vi "Update.vi"(6 "Table Name":string, 7 "condition":string, 8 "error in (no error)":errorcluster, 9 "Data List":variant, 10 "ColumnName List":variant, 11 "DataBase_SQL in":refnum<class "DataBase_SQL.lvclass">) -> (0 "error out":errorcluster, 2 "SQL Query":string, 3 "DataBase_SQL out":refnum<class "DataBase_SQL.lvclass">)   [LabVIEW 2021, in "DataBase_SQL.lvclass"]
uses:
  <userlib>/John_Lib/DataBase/DataBase_SQL/DataBase_SQL.lvclass
  <userlib>/John_Lib/DataBase/DataBase_SQL/DataBase_SQL.lvclass/DataBase_SQL.ctl
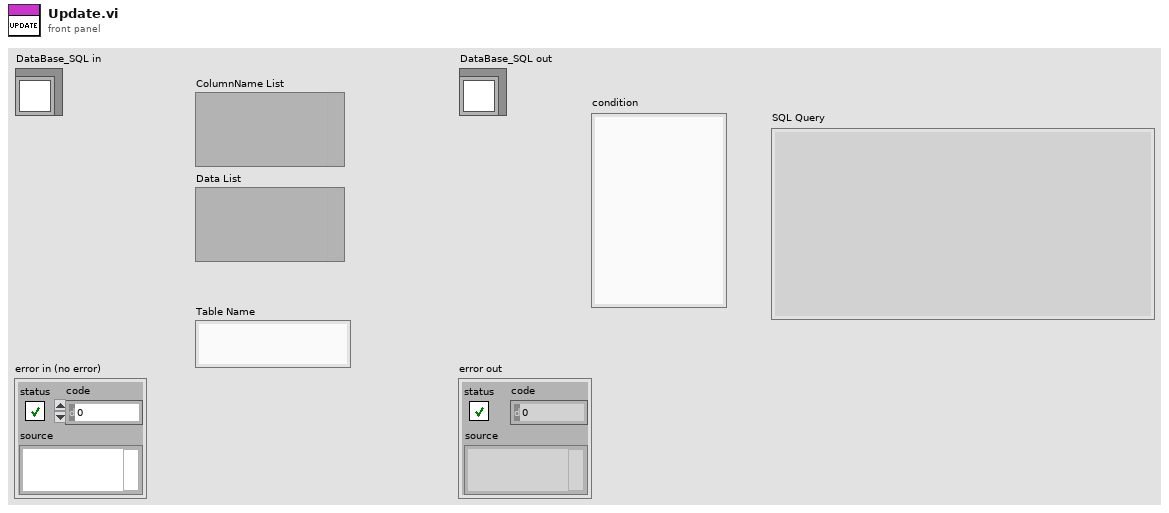
[diagram p1: front panel]
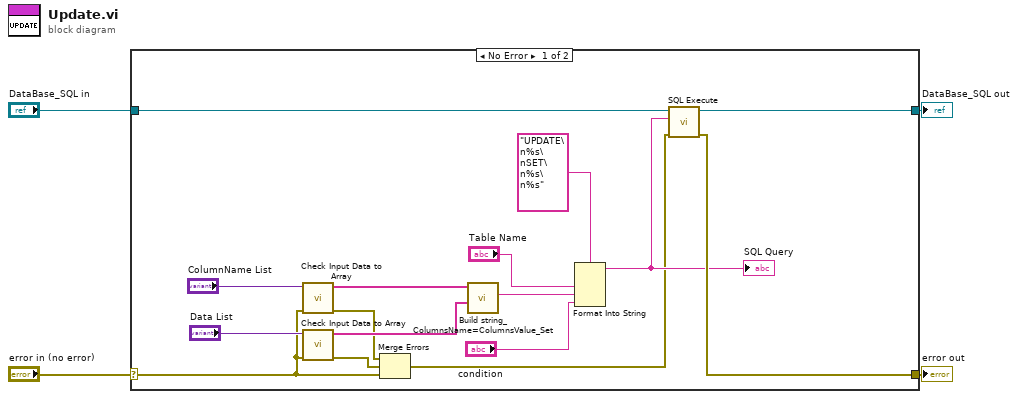
[diagram p0: block diagram]
diagram:
  n1 = case shown="No Error" "error in (no error)" {
    selector: "error in (no error)" -> [w8 w22]
    tunnel: [w16 w22] -> w3
    tunnel: [w18 w21] -> w1
    tunnel: "DataBase_SQL in" -> [w17 w21]
    frame No Error {
      n2 = call <userlib>:"Check Input Data to Array.vi"("error in (no error)"=w8, "String Array/ String"="ColumnName List") -> ("error out"=w6:errorcluster, "ColumnsNameList"=w11:string[])  [unwired: 8 in]
      n3 = call <userlib>:"Check Input Data to Array.vi"("error in (no error)"=w8, "String Array/ String"="Data List") -> ("error out"=w5:errorcluster, "ColumnsNameList"=w12:string[])  [unwired: 8 in]
      n4 = Merge Errors(w6, w5, w8) -> (w7:errorcluster)
      n5 = call <userlib>:"Build string_ColumnsName=ColumnsValue_Set.vi"("ColumnsValue"=w12, "ColumnsNameList"=w11) -> ("Total ColumnName='ColumnValue' String"=w20:string)  [unwired: 9 in]
      n6 = Format Into String(format string="UPDATE\n%s\nSET\n%s\n%s", "Table Name", w20, "condition") -> (resulting string=w13:string)  [unwired: 2 in, 1 out]
      "SQL Query" <- w13
      n7 = call-dynamic "SQL Execute.vi"("error in (no error)"=w7, "Command Text"=w13, "DataBase_SQL in"=w17) -> ("error out"=w16:errorcluster, "DataBase_SQL out"=w18:refnum<class "DataBase_SQL.lvclass">)  [unwired: 4 in, 3 out]
    }
    frame Error {
    }
  }
  "error out" <- w3
  "DataBase_SQL out" <- w1
